vi "Initialize OAuth for Slack.vi"(9 "Scopes":string[](array[string])=["users:read"], 10 "Client Secret":string, 11 "Client ID":string) -> (3 "Oauth2.Slack":refnum<class "Oauth2.Slack.lvclass">)   [LabVIEW 2013, in "Oauth2.Slack.lvclass"]
uses:
  Oauth2.Slack.lvclass
  Oauth2/Oauth2.lvclass
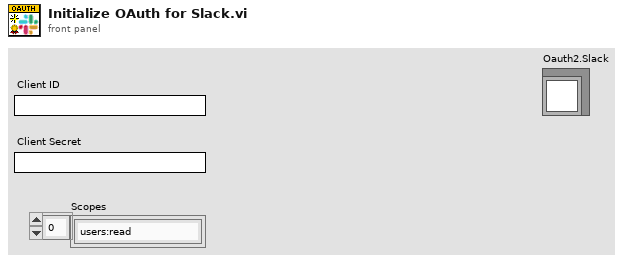
[diagram p1: front panel]
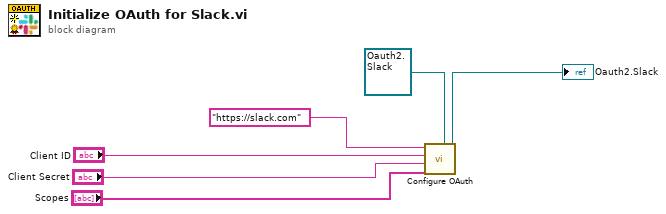
[diagram p0: block diagram]
diagram:
  n1 = call "Configure OAuth.vi"("Oauth2 in"=refnum<class "Oauth2.Slack.lvclass"> refnum ("Oauth2.GitHub in"), "scopes"="Scopes", "Client Secret"="Client Secret", "Client ID"="Client ID", "Authorization Server URI"="https://slack.com") -> ("Oauth2"=→"Oauth2.Slack":refnum<class "Oauth2.Slack.lvclass">)  [unwired: 5 in, 1 out]
